vi "ChemTrac read all (old).vi"(4 "State":i16, 5 "Time":dbl format="%.2f", 6 "Sensor Values":dbl[](array[numeric]), 7 "Set Points":dbl[](array[numeric])=[1.0, 3.0, 1.0]) -> (0 "required data":T2={"Set Point names"=["data interval (s)", "com port number", "device ID"], "required number of setpoints"=3, "required number of sensors"=0, "Sensor names"=[]}, 3 "output value":dbl)   [LabVIEW 2019]
uses:
  modbusrtu/MB buffer cmd.ctl
panel:
  out "error out":errorcluster
  in  "delay before write":u32=1000
  in  "Timeout":u32=600
  out "read":bool
  in  "Parity":u16(ring)=2 items=["None", "Odd", "Even", "Mark", "Space"]
  in  "set point inputs":T1
  # "Input Registers (Read Only)\nModbus Map: HydroAct 4 (75FC:4543:F24F:4856)\nAddress Size Type Device Description Ref.\n0 2 FLOAT UV-254 1.1 Official Value - UVA\n2 2 FLOAT UV-254 1.1 Official Value - UVT\n4 2 FLOAT UV-254 1.1 Official Value - Compensated UVA\n6 2 FLOAT UV-254 1.1 Official Value - COD\n8 2 FLOAT UV-254 1.1 Official Value - TOC\n10 2 FLOAT Particle Counter 1.2 Official Value - Cell\n12 2 FLOAT Particle Counter 1.2 Official Value - Laser\n14 2 FLOAT Particle Counter 1.2 Official Value - Total Counts\n16 2 FLOAT Particle Counter 1.2 Official Value - Counts Bin 1\n18 2 FLOAT Particle Counter 1.2 Official Value - Counts Bin 2\n20 2 FLOAT Particle Counter 1.2 Official Value - Counts Bin 3\n22 2 FLOAT Particle Counter 1.2 Official Value - Counts Bin 4\n24 2 FLOAT Particle Counter 1.2 Official Value - Counts Bin 5\n26 2 FLOAT Particle Counter 1.2 Official Value - Counts Bin 6\n28 2 FLOAT Particle Counter 1.2 Official Value - Total PPB\n30 2 FLOAT Particle Counter 1.2 Official Value - PPB Bin 1\n32 2 FLOAT Particle Counter 1.2 Official Value - PPB Bin 2\n34 2 FLOAT Particle Counter 1.2 Official Value - PPB Bin 3\n36 2 FLOAT Particle Counter 1.2 Official Value - PPB Bin 4\n38 2 FLOAT Particle Counter 1.2 Official Value - PPB Bin 5\n40 2 FLOAT Particle Counter 1.2 Official Value - PPB Bin 6\n42 2 FLOAT Particle Counter 1.3 Official Value - Cell\n44 2 FLOAT Particle Counter 1.3 Official Value - Laser\n46 2 FLOAT Particle Counter 1.3 Official Value - Total Counts\n48 2 FLOAT Particle Counter 1.3 Official Value - Counts Bin 1\n50 2 FLOAT Particle Counter 1.3 Official Value - Counts Bin 2\n52 2 FLOAT Particle Counter 1.3 Official Value - Counts Bin 3\n54 2 FLOAT Particle Counter 1.3 Official Value - Counts Bin 4\n56 2 FLOAT Particle Counter 1.3 Official Value - Counts Bin 5\n58 2 FLOAT Particle Counter 1.3 Official Value - Counts Bin 6\n60 2 FLOAT Particle Counter 1.3 Official Value - Total PPB\n62 2 FLOAT Particle Counter 1.3 Official Value - PPB Bin 1\n64 2 FLOAT Particle Counter 1.3 Official Value - PPB Bin 2\n66 2 FLOAT Particle Counter 1.3 Official Value - PPB Bin 3\n68 2 FLOAT Particle Counter 1.3 Official Value - PPB Bin 4\n70 2 FLOAT Particle Counter 1.3 Official Value - PPB Bin 5\n72 2 FLOAT Particle Counter 1.3 Official Value - PPB Bin 6"
  # "Enter the correct information for this control code in the required data structure below. Then make the current value default by right clicking on the border of the data structure. Select \"data operations\" and then select \"make current value default\". These values will be displayed by process controller."
  # "HydroACT has even parity by default."
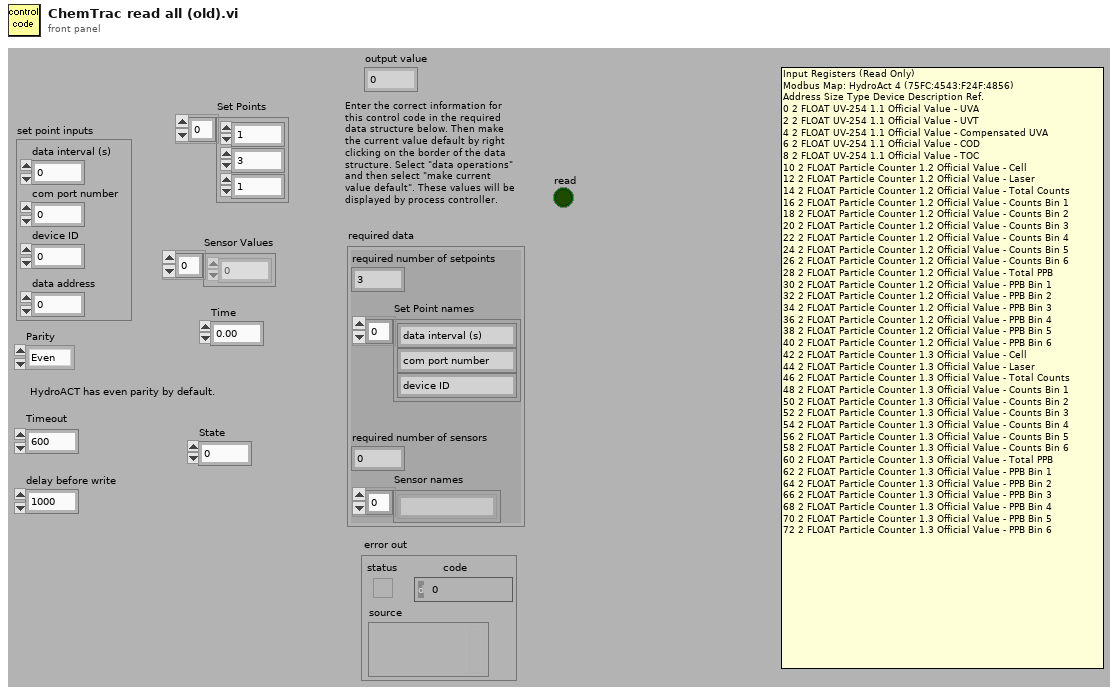
[diagram p1: front panel]
types:
  T1 = cluster{"data interval (s)":dbl, "com port number":u8, "device ID":u8, "data address":u8}
  T2 = cluster{"Set Point names":string[], "required number of setpoints":u8, "required number of sensors":u8, "Sensor names":string[]}
  T3 = cluster{"Set Points[0]":dbl, "Set Points[1]":dbl, "Set Points[2]":dbl}
  T4 = typedef "MB buffer cmd.ctl" = enum16{"Write", "Read", "Reset"}
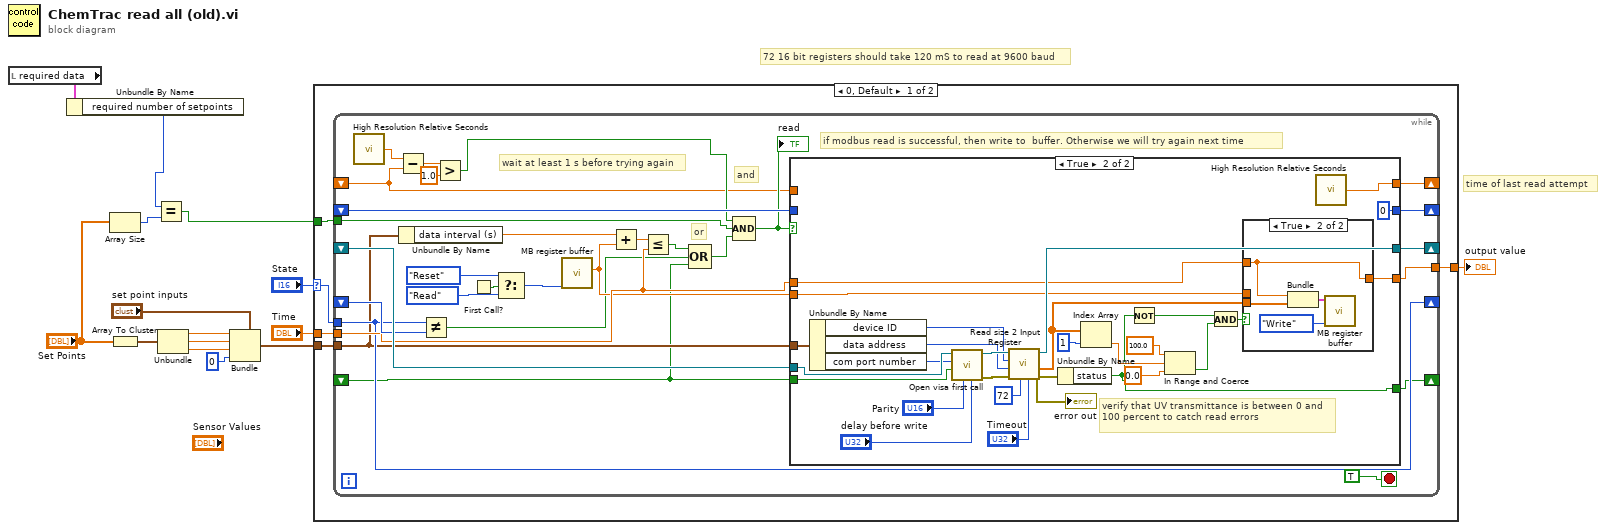
[diagram p0: block diagram]
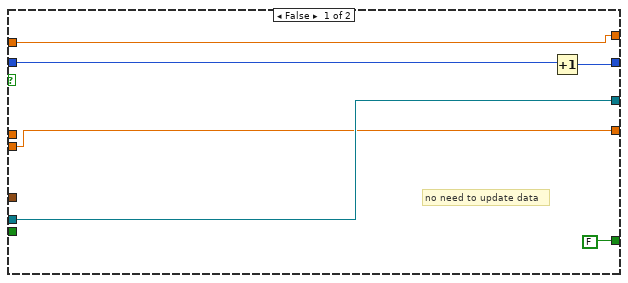
[diagram p2: hidden frame]
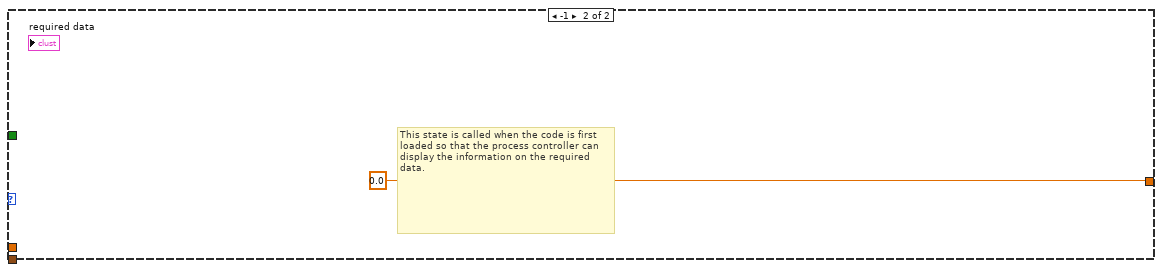
[diagram p4: hidden frame]
diagram:
  # "time of last read attempt"
  # "72 16 bit registers should take 120 mS to read at 9600 baud"
  n1 = local read "required data"() -> (w2:T2)
  n2 = Unbundle By Name(w2) -> ("required number of setpoints"=w1:u8)
  n3 = Array Size(array="Set Points") -> (size(s)=w4:i32)
  n4 = Array To Cluster(array="Set Points") -> (cluster=w12:T3)
  n5 = Equal?(x=w1, y=w4) -> (x = y?=w3:bool)
  n6 = Unbundle(w12) -> ("Set Points[0]"=w10:dbl, "Set Points[1]"=w13:dbl, "Set Points[2]"=w9:dbl)
  n7 = Bundle(cluster="set point inputs", "data interval (s)"=w10, "com port number"=w13, "device ID"=w9, "data address"=u8 0) -> (w8:T1)
  n8 = case shown="0, Default" "State" {
    selector: "State" -> [w18 _]
    tunnel: [w17 0.0 ("fraction on")] -> w14
    tunnel: w8 -> [w20 _]
    tunnel: "Time" -> [w19 _]
    tunnel: w3 -> [w16 _]
    frame 0, Default {
      n9 = while {
        shift-right: [w48] -> _
        shift-left: _ -> [w49]
        tunnel: w20 -> [w43]
        shift-right: [w35] -> _
        shift-left: _ -> [w27]
        shift-right: [w45] -> _
        shift-left: _ -> [w47]
        tunnel: w19 -> [w46]
        tunnel: w18 -> [w45]
        tunnel: [w41] -> w17
        tunnel: w16 -> [w33]
        shift-right: [w34] -> _
        shift-left: _ -> [w32]
        shift-right: [w26] -> _
        shift-left: _ -> [w21]
        stop <- TRUE stop-if-true
        # "wait at least 1 s before trying again"
        # "and"
        # "or"
        # "if modbus read is successful, then write to  buffer. Otherwise we will try again next time"
        n10 = call <vilib>:"High Resolution Relative Seconds.vi"() -> ("relative seconds"=w25:dbl)
        n11 = Subtract(x=w25, y=w21) -> (x-y=w24:dbl)
        n12 = Unbundle By Name(w43) -> ("data interval (s)"=w42:dbl)
        n13 = Not Equal?(x=w45, y=w47) -> (x != y?=w29:bool)
        n14 = Greater?(x=w24, y=1.0) -> (0:w22:bool)
        n15 = First Call?() -> (First Call?: T/F=w40:bool)
        n16 = Select(t=MB_buffer_cmd."Reset" ("command"), s=w40, f=MB_buffer_cmd."Read" ("command")) -> (s? t:f=w37:T4)
        n17 = call "MB register buffer.vi"("command"=w37) -> ("last read (s)"=w36:dbl)  [unwired: 9 in, 1 out]
        n18 = Add(x=w42, y=w36) -> (x+y=w44:dbl)
        n19 = Less Or Equal?(x=w44, y=w46) -> (x <= y?=w30:bool)
        n20 = Compound Arithmetic op=OR(w30, w29, w27) -> (w28:bool)
        n21 = Compound Arithmetic op=AND(w22, w33, w28) -> (w31:bool)
        "read" <- w31
        n22 = case shown="True" w31 {
          tunnel: w49 -> [w56 w84]
          tunnel: w27 -> [_ w76]
          tunnel: [w56 w83] -> w48
          tunnel: [FALSE ("status") w60] -> w35
          tunnel: w43 -> [_ w79]
          tunnel: w46 -> [_ w73]
          tunnel: [w55 w71] -> w41
          tunnel: w36 -> [w55 w70]
          tunnel: [w52 0] -> w34
          tunnel: w32 -> [w53 _]
          tunnel: [w51 w58] -> w26
          tunnel: w21 -> [w51 _]
          frame False {
            # "no need to update data"
            n23 = Increment(x=w53) -> (x+1=w52:i32)
          }
          frame True {
            # "verify that UV transmittance is between 0 and 100 percent to catch read errors"
            n24 = Unbundle By Name(w79) -> ("device ID"=w80:u8, "data address"=w78:u8, "com port number"=w77:u8)
            n25 = call "Open visa first call.vi"("delay before write"="delay before write", "Parity"="Parity", "error"=w76, "Com port"=w77, "VISA Refnum in"=w84) -> ("error out"=w81:errorcluster, "VISA Refnum out"=w82:refnum<visa-resource-name>)  [unwired: 5 in]
            n26 = call "Read size 2 Input Register.vi"("Timeout"="Timeout", "Quantity"=u16 72, "error in"=w81, "data address"=w78, "device ID"=w80, "VISA resource name"=w82) -> ("error out"=w64:errorcluster, "data array"=w69:sgl[], "VISA resource name out"=w83:refnum<visa-resource-name>)  [unwired: 1 in, 2 out]
            "error out" <- w64
            n27 = Unbundle By Name(w64) -> ("status"=w60:bool)
            n28 = Index Array(array=w69, index=1) -> (element=w67:sgl)
            n29 = Not(x=w60) -> (.not. x?=w62:bool)
            n30 = In Range and Coerce(upper limit=sgl 100.0, x=w67, lower limit=sgl 0.0) -> (In Range?=w63:bool)  [unwired: 1 out]
            n31 = And(x=w62, y=w63) -> (x .and. y?=w61:bool)
            n32 = case shown="True" w61 {
              tunnel: w69 -> [_ w89]
              tunnel: w73 -> [_ w86]
              tunnel: [w85 w86] -> w71
              tunnel: w70 -> [w85 _]
              frame False {
              }
              frame True {
                n33 = Bundle("Time"=w86, "data array"=w89) -> (w88:cluster{"Time":dbl, "data array":sgl[]})  [unwired: 1 in]
                n34 = call "MB register buffer.vi"("command"=MB_buffer_cmd."Write", "register array in"=w88) -> ()  [unwired: 8 in, 2 out]
              }
            }
            n35 = call <vilib>:"High Resolution Relative Seconds.vi"() -> ("relative seconds"=w58:dbl)
          }
        }
      }
    }
    frame -1 {
      # "This state is called when the code is first loaded so that the process controller can display the information on the required data."
    }
  }
  "output value" <- w14
